vi "Dashboard Main.vi"() -> ()   [LabVIEW 2015]
uses:
  <vilib>/Utility/miscctls.llb/LVRowAndColumnTypeDef.ctl
  <vilib>/event_ctls.llb/eventvkey.ctl
  <vilib>/Rock Robotics/WPI/Dashboard/WPI_DashboardLogging Global.vi
  <vilib>/Rock Robotics/Network Tables/NT Read Numeric Array.vi
  <vilib>/Utility/config.llb/Write Key (String).vi
  <vilib>/Utility/config.llb/Write Key (I32).vi
  <vilib>/Math Plots/2D Math Plots/2D Compass/2D Compass Datatype/Public/Plot Helper (Vector).vi
  <vilib>/Utility/config.llb/NI_LVConfig.lvlib
  <vilib>/Math Plots/2D Math Plots/2D Compass/2D Compass Datatype/2D Compass Datatype.lvclass
panel:
  out "Camera Image 2":T1(plugin-control)
  in  "Switch Cams":bool
  in  "TCP":refnum<k5>
  in  "Rec Mode":enum32{"Stop", "Record", "Playback"}(radio)
  in  "Vision":u16(ring) items=["Camera Off", "USB Camera SW", "USB Camera HW", "IP Camera"]
  out "Camera IP":string
  out "Image Message":string="Timeout in Camera Communications"
  in  "Dashboard Tab":T2(tab)
  out "Gyro":dbl(knob) scale=0.0..360.0
  in  "Select Auto":string(combo)="just over defense in front"
  out "NT Connection":bool
  in  "Camera Settings":T3={"Frame Rate"=30, "Compression"=30, "Size"=1} {"Frame Rate" scale=1.0..30.0; "Size" items=["640x480", "320x240", "160x120"]}
  out "MotorChart R":cluster{"Numeric":dbl, "Numeric":dbl}(graph)
  out "MotorChart L":T4(graph)
  out "MotorSliders R":cluster{"MotorSlide1":dbl, "MotorSlide2":dbl} {"MotorSlide2" scale=-1.0..1.0 scale format="%#_2e"; "MotorSlide1" scale=-1.0..1.0 scale format="%#_2e"}
  out "MotorSliders L":T5 {"MotorSlide4 2" scale=0.0..14.0 scale format="%#_2e"; "MotorSlide2" scale=-1.0..1.0 scale format="%#_2e"; "MotorSlide1" scale=-1.0..1.0 scale format="%#_2e"}
  out "JS1 Z":dbl(slide) scale=-1.0..1.0 scale format="%#_2e"
  out "JS1 Graph":cluster{"X":dbl, "Y":dbl}[](graph)
  out "JS1 Buttons":T6
  out "JS2 Z":dbl(slide) scale=-1.0..1.0 scale format="%#_2e"
  out "JS2 Graph":cluster{"X":dbl, "Y":dbl}[](graph)
  out "JS2 Buttons":T6
  out "Mode":T7(ring)=enum."Auto Disabled"
  in  "DB Camera Config":bool
  out "fps":dbl format="%#.1g"
  out "Mbps":dbl format="%#.1g"
  out "Mbps LED":bool
  in  "DB/String 9":string
  in  "DB/String 8":string
  in  "DB/String 7":string
  in  "DB/String 6":string
  in  "DB/String 5":string
  in  "DB/String 4":string
  in  "DB/String 3":string
  in  "DB/String 2":string
  in  "DB/String 1":string
  in  "DB/String 0":string
  in  "DB/Slider 0":dbl(slide) scale=0.0..5.0
  in  "DB/Slider 1":dbl(slide) scale=0.0..5.0
  in  "DB/Slider 2":dbl(slide) scale=0.0..5.0
  in  "DB/Slider 3":dbl(slide) scale=0.0..5.0
  out "DB/LED 3":bool
  out "DB/LED 2":bool
  out "DB/LED 1":bool
  out "DB/LED 0":bool
  in  "DB/Button 3":bool
  in  "DB/Button 2":bool
  in  "DB/Button 1":bool
  in  "DB/Button 0":bool caption="New Name"
  in  "AutoMode":dbl
  in  "ClawUPDownSensitivity":dbl(slide)=0.45 step=0.025 scale=0.0..1.0
  in  "HookSensitivity":dbl(slide)=0.1 step=0.025 scale=0.0..1.0
  in  "ElevatorSensitivity":dbl(slide)=0.8500000000000001 step=0.025 scale=0.0..1.0
  in  "ClappySensitivity":dbl(slide)=0.8500000000000001 step=0.025 scale=0.0..1.0
  in  "Elevator Encoder Re-Set":bool
  in  "Elevator Height":dbl(slide) scale=0.0..7.0
  out "Manual Enabled":bool
  out "Joystick Invert":bool
  in  "F/B Invert":bool
  in  "TurningSensitivity":dbl(slide)=0.75 step=0.025 scale=0.0..1.0
  in  "ForwardSensitivity":dbl(slide)=0.8500000000000001 step=0.025 scale=0.0..1.0
  in  "Test Slider":dbl(slide) scale=0.0..100.0 scale format="%#_3g"
  in  "On/Off":bool caption="Solenoid"
  in  "Test Name":u16(ring) items=["Select the test to run..."]
  in  "Test Tree":string(tree)
  in  "Motor":cluster{"Value":dbl, "Enable":bool} {"Value" scale=-1.0..1.0 scale format="%#_3g"}
  out "Progress":T8 {"Test Progress" scale=0.0..100.0}
  in  "Rev/Fwd":cluster{"Forward":bool, "Reverse":bool}
  in  "Test Ring":u16(ring) items=["Monochrome", "Color"]
  out "Cmd Status":string
  in  "Execute Command":bool
  in  "Command Params":string[][](table)
  in  "Command Selection":i32(listbox)
  in  "CheckList":i32(listbox)
  out "Tree":string(tree)
  out "Camera Image":T1(plugin-control)
  out "Background":bool
  # "Left"
  # "Front"
  # "Right"
  # "Battery"
  # "If both inverted,\n it isn't inverted"
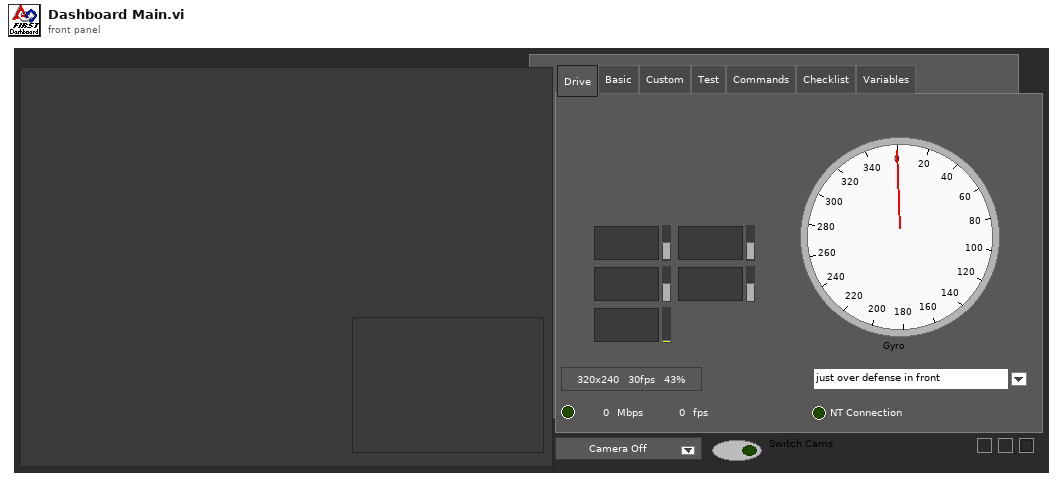
[diagram p1: front panel]
types:
  T1 = typedef "IMAQ Image.ctl" = refnum<image>
  T2 = enum32{"Drive", "Basic", "Custom", "Test", "Commands", "Checklist", "Variables"}
  T3 = cluster{"Frame Rate":i32, "Compression":i32, "Size":u16}
  T4 = cluster{"Numeric":dbl, "Numeric":dbl, "Battery V":dbl}
  T5 = cluster{"MotorSlide1":dbl, "MotorSlide2":dbl, "MotorSlide4 2":dbl}
  T6 = cluster{bool, bool, bool, bool, bool, bool, bool, bool, bool, bool, bool, bool}
  T7 = enum8{"Tele-Op Disabled", "Tele-Op Enabled", "Auto Disabled", "Auto Enabled", "Test Disabled", "Test Enabled", "Disconnected", "No Code", "E-Stop"}
  T8 = cluster{"Test Progress":u8, "Test Progress Text":string}
  T9 = typedef "Image Type" = u32
  T10 = cluster{"IDs":cluster{"RPC field ID":u16, "Unique ID":u16}, "String":string}
  T11 = enum32{"Drive", "Basic", "Custom", "Test", "Checklist", "Variables"}
  T12 = cluster{"Camera Image":refnum<vi>, "Dashboard Tab":refnum<vi>, "Background":refnum<vi>, "Vision":refnum<vi>, "Rec Mode":refnum<vi>, "Test Slider":refnum<vi>, "On/Off ":refnum<vi>, "Test Ring":refnum<vi>, "Rev/Fwd":refnum<vi>, "Test Name":refnum<vi>, "Motor":refnum<vi>, "Progress":refnum<vi>, "CheckList":refnum<vi>, "Tree":refnum<vi>, "Test Tree":refnum<vi>, "Command Params":refnum<vi>, "Command Selection":refnum<vi>, "Execute Command":refnum<vi>, "Cmd Status":refnum<vi>}
  T13 = cluster{"Error Strings":string, "Disable Counts":cluster{u16, u16}, "Rail Faults":cluster{u16, u16, u16}, "Robot IP":string, "DB Mode":u8, "Event Info":cluster{"Name":string, "Type":u8, "Number":u16, "Replay":u8}, "Camera Addr":string}
  T14 = cluster{"Storage":cluster{"Disk Free":u64, "RAM Block":u32, "RAM free":u32}, "CPU Utilization":cluster{"CPU % ISR":sgl, "CPU % Time Crit":sgl, "CPU % Timed Str":sgl, "CPU % High":sgl, "CPU % Above":sgl, "CPU % Normal":sgl, "CPU % Low":sgl}, "CAN":cluster{"% Bus Utilization":sgl, "Bus Off Cnt":u32, "TX_FIFO Full Cnt":u32, "Receive Error Cnt":u8, "Transmit Error Cnt":u8}, "HID":cluster{"HID Outputs":u32, "Rumble Low":u16, "Rumble High":u16}[]}
  T15 = cluster{"Status bits":cluster{"Test Mode":bool, "Autonomous":bool, "Enabled":bool, "Code Start":bool, "Brownout":bool, "Reserved 2":bool, "Reserved 3":bool, "E-Stop":bool}, "Code Trace":cluster{"Disabled":bool, "TeleOp":bool, "Auto":bool, "Test":bool}, "Controller Type":enum16{"unknown", "cRIO", "roboRio"}, "Code?":enum16{"unknown", "noCode", "code"}, "Battery V":dbl}
  T16 = cluster{"Control Bits":cluster{"TestMode":bool, "Autonomous":bool, "Enabled":bool, "FMS Present":bool, bool, bool, bool, "E-Stop":bool}, "Team Station ":u8, "Countdown":sgl, "Joystick Values":cluster{"Axes":dbl[], "Buttons":bool[], "POVs":i16[]}[]}
  T17 = cluster{"Axes":dbl[], "Buttons":bool[], "POVs":i16[]}[]
  T18 = cluster{"Axes":dbl[], "Buttons":bool[], "POVs":i16[]}
  T19 = cluster{"Buttons[0]":bool, "Buttons[1]":bool, "Buttons[2]":bool, "Buttons[3]":bool, "Buttons[4]":bool, "Buttons[5]":bool, "Buttons[6]":bool, "Buttons[7]":bool, "Buttons[8]":bool, "Buttons[9]":bool, "Buttons[10]":bool, "Buttons[11]":bool}
  T20 = typedef "NI_LVConfig.lvlib/Config Data RefNum.ctl" = refnum<k1>
  T21 = cluster{"Operation":enum16{"Update", "Clear"}, "Color Box":u32}[]
  T22 = typedef "eventvkey.ctl" = enum16{"ASCII", "Enter", "Return", "Shift", "Ctrl", "Alt", "Cmd", "Opt", "Caps", "NumLock", "Clear", "Break", "Up", "Down", "Left", "Right", "Insert", "Delete", "Home", "End", "PageUp", "PageDown", "Escape", "Help", "Pause", "ScrollLock", "F1", "F2", "F3", "F4", "F5", "F6", "F7", "F8", "F9", "F10", "F11", "F12", "F13", "F14", "F15", "F16", "F17", "F18", "F19", "F20", "F21", "F22", "F23", "F24", "Play", "VolumeUp", "VolumeDown", "Mute", "Two Byte Char"}
  T23 = cluster{"Image Size":bool, "Image Type":bool, "Pixel Value":bool, "ROI Information":bool, "Zoom Factor":bool}
  T24 = enum8{"Enabled", "Disabled", "Disabled and Grayed Out"}
  T25 = cluster{"Operation":enum16{"Update", "Clear"}, "Color Box":u32}
  T26 = typedef "LVRowAndColumnTypeDef.ctl" = cluster{"Row":i32, "Column":i32}
  T27 = cluster{"Shift":bool, "Ctrl":bool, "Alt":bool, "Cmd":bool, "Opt":bool}
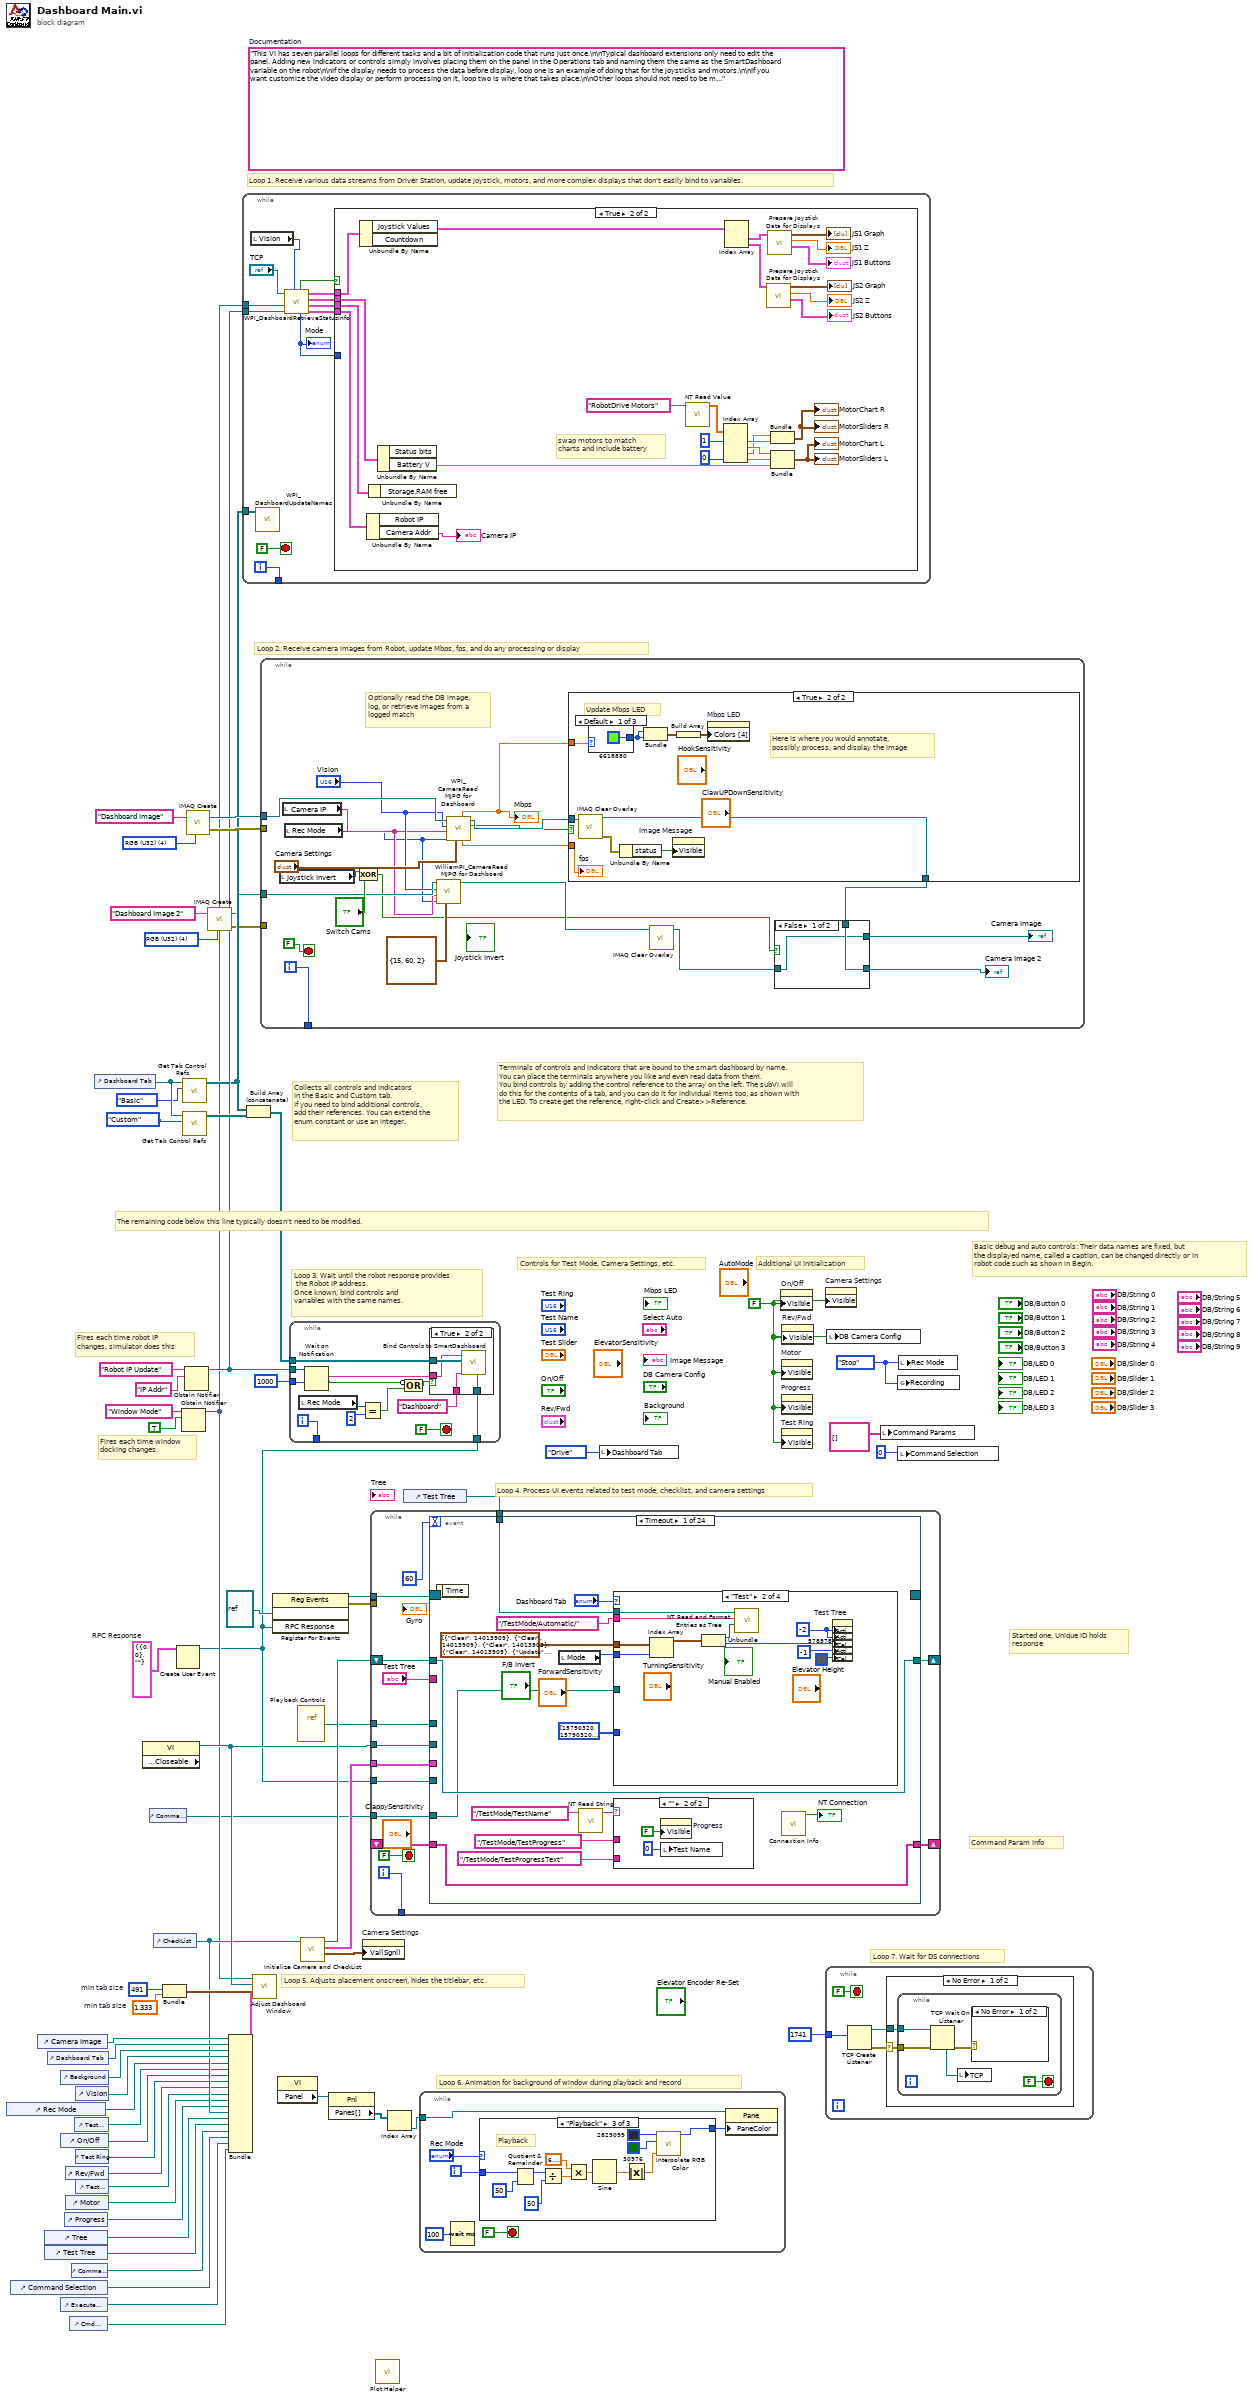
[diagram p0: block diagram]
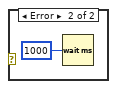
[diagram p2: hidden frame]
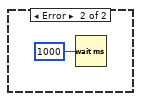
[diagram p3: hidden frame]
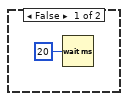
[diagram p4: hidden frame]
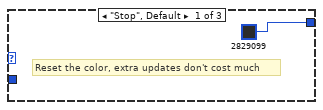
[diagram p5: hidden frame]
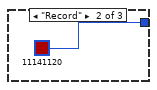
[diagram p6: hidden frame]
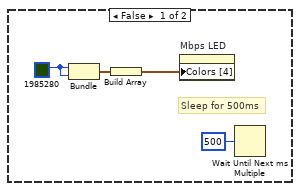
[diagram p9: hidden frame]
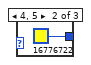
[diagram p10: hidden frame]
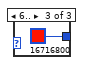
[diagram p11: hidden frame]
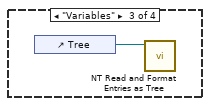
[diagram p13: hidden frame]
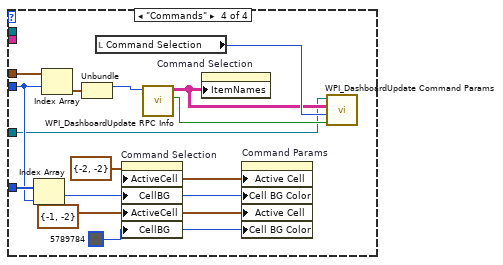
[diagram p14: hidden frame]
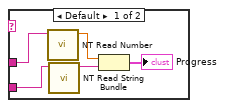
[diagram p15: hidden frame]
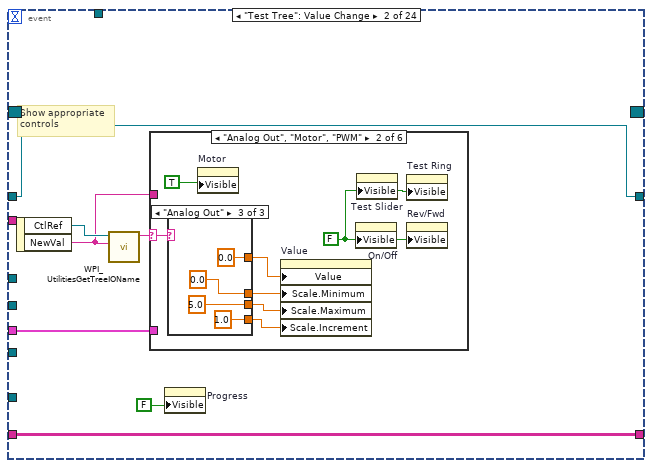
[diagram p16: hidden frame]
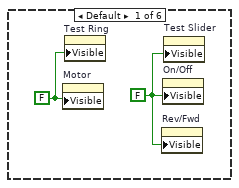
[diagram p17: hidden frame]
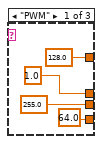
[diagram p18: hidden frame]
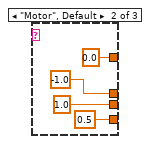
[diagram p19: hidden frame]
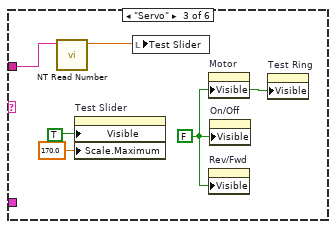
[diagram p20: hidden frame]
diagram:
  w4 = T9 4 items=["Grayscale (U8)", "Grayscale (I16)", "Grayscale (SGL)", "Complex (CSG)", "RGB (U32)", "HSL (U32)", "RGB (U64)"] ("Image Type")
  w11 = T10 {"IDs"={"RPC field ID"=0, "Unique ID"=0}, "String"=""}  # RPC Response
  w37 = 491  # min tab size
  w36 = 1.333  # min tab size
  w45 = enum32{"Stop", "Record", "Playback"}."Stop" ("Rec Mode")
  w19 = FALSE ("Visible")
  (unwired) "This VI has seven parallel loops for different tasks and a bit of initialization code that runs just once.\n\nTypical dashboard extensions only need to edit the panel. Adding new indicators or controls simply involves placing them on the panel in the Operations tab and naming them the same as the SmartDashboard variable on the robot\n\nIf the display needs to process the data before display, loop one is an example of doing that for the joysticks and motors.\n\nIf you want customize the video display or perform processing on it, loop two is where that takes place.\n\nOther loops should not need to be modified. They are pretty standard, and document the task they perform."  # Documentation
  w65 = T9 4 items=["Grayscale (U8)", "Grayscale (I16)", "Grayscale (SGL)", "Complex (CSG)", "RGB (U32)", "HSL (U32)", "RGB (U64)"] ("Image Type")
  # "Command Param Info"
  # "Started one, Unique ID holds\nresponse"
  # "Loop 7. Wait for DS connections"
  # "Basic debug and auto controls: Their data names are fixed, but\nthe displayed name, called a caption, can be changed directly or in\nrobot code such as shown in Begin."
  # "Controls for Test Mode, Camera Settings, etc."
  # "Additional UI Initialization"
  # "Loop 6. Animation for background of window during playback and record"
  # "Fires each time robot IP\nchanges, simulator does this"
  # "Fires each time window\ndocking changes."
  # "Collects all controls and indicators\nin the Basic and Custom tab.\nIf you need to bind additional controls,\nadd their references. You can extend the\nenum constant or use an integer."
  # "The remaining code below this line typically doesn't need to be modified."
  # "Loop 4. Process UI events related to test mode, checklist, and camera settings"
  # "Terminals of controls and indicators that are bound to the smart dashboard by name.\nYou can place the terminals anywhere you like and even read data from them.\nYou bind controls by adding the control reference to the array on the left. The subVI will\ndo this for the contents of a tab, and you can do it for individual items too, as shown with\nthe LED. To create get the reference, right-click and Create>>Reference."
  # "Loop 3. Wait until the robot response provides\n the Robot IP address.\nOnce known, bind controls and\nvariables with the same names."
  # "Loop 5. Adjusts placement onscreen, hides the titlebar, etc."
  # "Loop 1. Receive various data streams from Driver Station, update joystick, motors, and more complex displays that don't easily bind to variables."
  # "Loop 2. Receive camera images from Robot, update Mbps, fps, and do any processing or display"
  n1 = control-ref of="Rec Mode"() -> (w25:refnum<vi>)
  n2 = control-ref of="Command Selection"() -> (w10:refnum<vi>)
  n3 = control-ref of="Camera Image"() -> (w40:refnum<vi>)
  n4 = control-ref of="Tree"() -> (w29:refnum<vi>)
  n5 = control-ref of="Test Tree"() -> (w28:refnum<vi>)
  n6 = control-ref of="Dashboard Tab"() -> (w39:refnum<vi>)
  n7 = control-ref of="Execute Command"() -> (w12:refnum<vi>)
  n8 = control-ref of="Background"() -> (w34:refnum<vi>)
  n9 = control-ref of="On/Off"() -> (w23:refnum<vi>)
  n10 = control-ref of="Progress"() -> (w20:refnum<vi>)
  n11 = control-ref of="Rev/Fwd"() -> (w21:refnum<vi>)
  n12 = control-ref of="Motor"() -> (w26:refnum<vi>)
  n13 = control-ref of="Cmd Status"() -> (w6:refnum<vi>)
  n14 = control-ref of="Command Params"() -> (w13:refnum<vi>)
  n15 = control-ref of="Test Slider"() -> (w24:refnum<vi>)
  n16 = control-ref of="Vision"() -> (w38:refnum<vi>)
  n17 = control-ref of="Test Ring"() -> (w22:refnum<vi>)
  n18 = control-ref of="Test Name"() -> (w27:refnum<vi>)
  n19 = control-ref of="Dashboard Tab"() -> (w43:refnum<vi>)
  n20 = property class="VI" props=["Front Panel.Closeable"]() -> (reference out=w44:refnum<vi>)  [unwired: 2 in, 2 out]
  n21 = control-ref of="Command Params"() -> (w5:refnum<vi>)
  n22 = control-ref of="CheckList"() -> (w30:refnum<vi>)
  n23 = Bundle("min tab size"=w37, "min tab size"=w36) -> (w35:cluster{"min tab size":i32, "min tab size":dbl})  [unwired: 1 in]
  n24 = Create User Event(user event datatype=w11) -> (user event=w7:refnum<user-event>)  [unwired: 1 in, 1 out]
  n25 = Obtain Notifier(name (unnamed)="Window Mode", notification data type=TRUE) -> (notifier out=w16:refnum<notifier>)  [unwired: 2 in, 2 out]
  n26 = call <vilib>:"Get Tab Control Refs.vi"("Page Index"=T11."Basic" ("Dashboard Tab"), "TabControl in"=w43) -> ("ControlsOnPage"=w17:refnum<vi>[])  [unwired: 9 in]
  n27 = call <vilib>:"Get Tab Control Refs.vi"("Page Index"=T11."Custom" ("Dashboard Tab"), "TabControl in"=w43) -> ("ControlsOnPage"=w42:refnum<vi>[])  [unwired: 9 in]
  n28 = Obtain Notifier(name (unnamed)="Robot IP Update", notification data type="IP Addr" ("name (unnamed)")) -> (notifier out=w18:refnum<notifier>)  [unwired: 2 in, 2 out]
  n29 = call "IMAQ Create"("Image Name"="Dashboard Image", "Image Type"=w65) -> ("New Image"=w63:T1, "error out"=w62:errorcluster)  [unwired: 2 in, 1 out]
  n30 = call "IMAQ Create"("Image Name"="Dashboard Image 2", "Image Type"=w4) -> ("New Image"=w2:T1, "error out"=w1:errorcluster)  [unwired: 2 in, 1 out]
  n31 = Bundle("Camera Image"=w40, "Dashboard Tab"=w39, "Background"=w34, "Vision"=w38, "Rec Mode"=w25, "Test Slider"=w24, "On/Off"=w23, "Test Ring"=w22, "Rev/Fwd"=w21, "Test Name"=w27, "Motor"=w26, "Progress"=w20, "CheckList"=w30, "Tree"=w29, "Test Tree"=w28, "Command Params"=w13, "Command Selection"=w10, "Execute Command"=w12, "Cmd Status"=w6) -> (w31:T12)  [unwired: 1 in]
  n32 = while {
    tunnel: [w77] -> _
    tunnel: w18 -> [w71]
    tunnel: w17 -> [w70]
    tunnel: w16 -> [w66]
    i -> [w77]
    stop <- FALSE stop-if-true
    n33 = local read "Vision"() -> (w68:u16)
    n34 = call <vilib>:"WPI_DashboardUpdateNames.vi"("Controls on Tab"=w70) -> ()  [unwired: 11 in]
    n35 = call <vilib>:"WPI_DashboardRetrieveStatusInfo.vi"("Vision"=w68, "Binding Refnum"=w71, "Window Mode Notifier"=w66, "TCP Cnx"="TCP") -> ("Power and Errors"=w72:T13, "Robot Metrics"=w75:T14, "Status Info"=w76:T15, "Control Info"=w73:T16, "Robot Mode"=w69:T7, "Process?"=w74:bool)  [unwired: 2 in]
    "Mode" <- w69
    n36 = case shown="True" w74 {
      tunnel: w76 -> [_ w104]
      tunnel: w75 -> [_ w103]
      tunnel: w73 -> [_ w102]
      tunnel: w72 -> [_ w101]
      tunnel: w69 -> [_ _]
      frame False {
        n37 = Wait (ms)(milliseconds to wait=u32 20) -> ()  [unwired: 1 out]
      }
      frame True {
        # "swap motors to match\ncharts and include battery"
        n38 = Unbundle By Name(w102) -> ("Joystick Values"=w91:T17)  [unwired: 1 out]
        n39 = Unbundle By Name(w101) -> ("Camera Addr"=→"Camera IP":string)  [unwired: 1 out]
        n40 = Unbundle By Name(w103) -> ()  [unwired: 1 out]
        n41 = Unbundle By Name(w104) -> ("Battery V"=w92:dbl)  [unwired: 1 out]
        n42 = call-poly <vilib>:"NT Read Value.vi"("Name"="RobotDrive Motors") -> ("Numeric Array"=w80:dbl[])  [unwired: 9 in, 1 out]
        n43 = Index Array(array=w80, index #1=1, index #4=0) -> (element #1=w96:dbl, element #2=w97:dbl, element #3=w95:dbl, element #4=w100:dbl)  [unwired: 2 in]
        n44 = Index Array(array=w91) -> (element #1=w90:T18, element #2=w85:T18)  [unwired: 2 in]
        n45 = call "Prepare Joystick Data for Displays.vi"("Joystick Values"=w85) -> ("Buttons"=→"JS2 Buttons":T19, "Z Axis"=→"JS2 Z":dbl, "Cartesian Data"=→"JS2 Graph":cluster{"X axis":dbl, "X axis":dbl}[])  [unwired: 8 in]
        n46 = call "Prepare Joystick Data for Displays.vi"("Joystick Values"=w90) -> ("Buttons"=→"JS1 Buttons":T19, "Z Axis"=→"JS1 Z":dbl, "Cartesian Data"=→"JS1 Graph":cluster{"X axis":dbl, "X axis":dbl}[])  [unwired: 8 in]
        n47 = Bundle("Numeric"=w95, "Numeric"=w96) -> (→"MotorChart R" →"MotorSliders R":cluster{"Numeric":dbl, "Numeric":dbl})  [unwired: 1 in]
        n48 = Bundle("Numeric"=w97, "Numeric"=w100, "Battery V"=w92) -> (→"MotorChart L" →"MotorSliders L":T4)  [unwired: 1 in]
      }
    }
  }
  n49 = Build Array (concatenate)(w17, w42) -> (w41:refnum<vi>[])
  n50 = call "Adjust Dashboard Window.vi"("Sizing Refnums"=w31, "Size Constraints"=w35, "VI"=w44, "WIn Mode"=w16) -> ()  [unwired: 8 in]
  n51 = while {
    tunnel: w63 -> [w123]
    tunnel: w62 -> [_]
    tunnel: [w124] -> _
    tunnel: w2 -> [w109]
    tunnel: w1 -> [_]
    i -> [w124]
    stop <- FALSE stop-if-true
    # "Optionally read the DB image,\nlog, or retrieve images from a\nlogged match"
    n52 = local read "Joystick Invert"() -> (w116:bool)
    n53 = local read "Camera IP"() -> (w107:string)
    n54 = local read "Rec Mode"() -> (w106:enum32{"Stop", "Record", "Playback"})
    n55 = Exclusive Or(1:"Switch Cams", 2:w116) -> (0:w105:bool)
    n56 = call "WilliamPI_CameraRead MJPG for Dashboard.vi"("Camera Settings"=T3 {"Frame Rate"=15, "Compression"=60, "Size"=2}, "Rec Mode"=w106, "Camera IP"=w107, "Camera Mode"="Vision", "Refnum in"=w109) -> ("Refnum out"=w113:T1)  [unwired: 3 in, 3 out]
    n57 = call <vilib>:"WPI_CameraRead MJPG for Dashboard.vi"("Camera Settings"="Camera Settings", "Rec Mode"=w106, "Camera IP"=w107, "Camera Mode"="Vision", "Refnum in"=w123) -> ("Active"=w117:bool, "Refnum out"=w119:T1, "FPS"=w121:dbl, "Bandwidth (Mbps)"=w120:dbl)  [unwired: 3 in]
    "Mbps" <- w120
    n58 = case shown="True" w117 {
      tunnel: w121 -> [_ w137]
      tunnel: w120 -> [_ w136]
      tunnel: w119 -> [_ w135]
      tunnel: [_ w134] -> w115
      frame False {
        w130 = u32 1985280 ("Color Box")
        # "Sleep for 500ms"
        n59 = Bundle("Color Box"=w130, "Color Box"=w130) -> (w132:cluster{"Color Box":u32, "Color Box":u32})  [unwired: 1 out]
        n60 = Build Array(w132) -> (w131:cluster{"Color Box":u32, "Color Box":u32}[])
        n61 = property on="Mbps LED" class="Bool (strict)"("Colors [4]"=w131) -> ()  [unwired: 2 in, 2 out]
        n62 = Wait Until Next ms Multiple(millisecond multiple=u32 500) -> ()  [unwired: 1 out]
      }
      frame True {
        # "Here is where you would annotate,\npossibly process, and display the image"
        # "Update Mbps LED"
        n63 = call "IMAQ Clear Overlay"("Image"=w135) -> ("error out"=w141:errorcluster, "Image Out"=w134:T1)  [unwired: 2 in, 7 out]
        n64 = case shown="Default" w136 {
          tunnel: [u32 6618880 ("Color Box") u32 16776722 ("Color Box") u32 16716800 ("Color Box")] -> w138
          frame Default {
          }
          frame 4, 5 {
          }
          frame 6.. {
          }
        }
        n65 = Unbundle By Name(w141) -> ("status"=w142:bool)
        n66 = Bundle("Color Box"=w138, "Color Box"=w138) -> (w140:cluster{"Color Box":u32, "Color Box":u32})  [unwired: 1 out]
        n67 = property on="Image Message" class="Str"("Visible"=w142) -> ()  [unwired: 2 in, 2 out]
        n68 = Build Array(w140) -> (w139:cluster{"Color Box":u32, "Color Box":u32}[])
        n69 = property on="Mbps LED" class="Bool (strict)"("Colors [4]"=w139) -> ()  [unwired: 2 in, 2 out]
        "fps" <- w137
      }
    }
    n70 = call "IMAQ Clear Overlay"("Image"=w113) -> ("Image Out"=w112:T1)  [unwired: 2 in, 8 out]
    n71 = case shown="False" w105 {
      tunnel: w115 -> [w127 w129]
      tunnel: [w126 w129] -> w114
      tunnel: w112 -> [w126 w128]
      tunnel: [w127 w128] -> w111
      frame False {
      }
      frame True {
      }
    }
    "Camera Image" <- w114
    "Camera Image 2" <- w111
  }
  n72 = register-events(refnum<vi> refnum, w7) -> (reference out=w49:refnum<event-registration>, error out=w48:errorcluster)  [unwired: 2 in]
  n73 = property class="VI"() -> ("Panel"=w52:refnum<vi>)  [unwired: 2 in, 2 out]
  n74 = while {
    tunnel: w41 -> [w158]
    tunnel: w18 -> [w156]
    tunnel: [w154] -> _
    tunnel: u32 1000 ("milliseconds to wait") -> [w153]
    tunnel: w7 -> [w146]
    i -> [w154]
    stop <- FALSE stop-if-true
    n75 = local read "Rec Mode"() -> (w149:enum32{"Stop", "Record", "Playback"})
    n76 = Wait on Notification(notifier=w156, timeout in ms (-1)=w153) -> (notification=w155:string, timed out?=w151:bool)  [unwired: 2 in, 2 out]
    n77 = Equal?(x=w149, y=u16 2 ("Rec Mode")) -> (x = y?=w150:bool)
    n78 = Compound Arithmetic op=OR(invert w151, w150) -> (w152:bool)
    n79 = case shown="True" w152 {
      tunnel: w158 -> [_ w162]
      tunnel: w155 -> [_ w161]
      tunnel: "Dashboard" -> [_ w160]
      tunnel: w146 -> [_ w159]
      frame False {
      }
      frame True {
        n80 = call <vilib>:"Bind Controls to SmartDashboard.vi"("RPC ref"=w159, "Client Name"=w160, "Bound Control Refs"=w162, "Server IP Address"=w161) -> ()  [unwired: 8 in]
      }
    }
  }
  n81 = vi-ref "Playback Controls.vi"() -> (w50:refnum<vi>)
  n82 = call "Initialize Camera and CheckList.vi"("ListBox in"=w30) -> ("Cluster"=w56:cluster{"value":i32, "value":i32, "index":i32}, "Array"=w57:cluster{string[]}[], "File Refnum"=w55:T20)  [unwired: 8 in]
  n83 = property class="Pnl"(reference=w52) -> ("Panes[]"=w53:refnum<vi>[])  [unwired: 1 in, 2 out]
  n84 = property on="Camera Settings" class="Clust (strict)"("Val(Sgnl)"=w56) -> ()  [unwired: 2 in, 2 out]
  n85 = call-poly <vilib>:"Plot Helper.vi"() -> ()  [unwired: 4 in, 8 out]
  n86 = Index Array(array=w53) -> (element=w51:refnum<vi>)  [unwired: 1 in]
  n87 = control-ref of="Test Tree"() -> (w54:refnum<vi>)
  n88 = while {
    tunnel: w57 -> [w174]
    shift-right: [w173] -> _
    shift-left: w55 -> [w172]
    tunnel: [w171] -> _
    tunnel: w54 -> [w170]
    tunnel: w50 -> [w169]
    tunnel: w49 -> [w168]
    tunnel: w48 -> [_]
    tunnel: w44 -> [w167]
    tunnel: w7 -> [w166]
    tunnel: w5 -> [w165]
    shift-right: [w164] -> _
    shift-left: _ -> [w163]
    i -> [w171]
    stop <- FALSE stop-if-true
    n89 = event shown="[0] Timeout" {
      selector: w168 -> [_ _ _ _ _ _ _ _ _ _ _ _ _ _ _ _ _ _ _ _ _ _ _ _]
      dyn-events: [_ _ _ _ _ _ _ _ _ _ _ _ _ _ _ _ _ _ w483 _ _ _ _ _] -> _
      timeout: u32 60 ("milliseconds to wait") -> [_ _ _ _ _ _ _ _ _ _ _ _ _ _ _ _ _ _ _ _ _ _ _ _]
      tunnel: w170 -> [w187 _ _ _ _ _ _ _ _ _ _ _ _ _ _ _ _ _ _ _ _ _ _ _]
      tunnel: "Test Tree" -> [_ _ _ _ _ _ _ _ _ _ _ _ _ w446 w455 w458 w463 w472 _ _ _ _ _ _]
      tunnel: w174 -> [_ w225 _ _ _ _ _ _ _ _ _ w408 w439 _ _ _ _ _ _ _ _ _ _ _]
      tunnel: [w184 w224 w328 w334 w344 w348 w354 w366 w374 w380 w393 w407 w432 w445 w453 w457 w462 w471 w485 w501 w503 w511 w522 w527] -> w173
      tunnel: w172 -> [w184 w224 w328 w334 w344 w348 w354 w366 w374 w380 w393 w406 w432 w445 w453 w457 w462 w471 w485 w501 w503 w511 w522 w527]
      tunnel: w169 -> [_ _ _ _ _ _ _ _ _ _ _ _ _ _ _ _ _ _ w486 _ w506 _ _ _]
      tunnel: w167 -> [_ _ _ _ _ _ _ _ _ _ _ _ _ _ _ _ _ _ w481 _ _ _ _ _]
      tunnel: w166 -> [_ _ _ _ _ _ _ _ _ _ _ _ _ _ _ _ _ _ w477 _ _ _ _ _]
      tunnel: w165 -> [w179 _ _ _ _ _ w352 _ _ _ _ _ _ _ _ _ _ _ _ _ _ _ _ _]
      tunnel: [w178 w223 w327 w333 w343 w349 w350 w360 w371 w379 w392 w405 w431 w444 w452 w456 w461 w470 w476 w499 w502 w507 w515 w528] -> w164
      tunnel: w163 -> [w178 w223 w327 w333 w343 w349 w350 _ _ w379 w392 w405 w431 w444 w452 w456 w461 w470 w476 w499 w502 w507 w515 w528]
      event Timeout {
        n90 = event-data() -> ()  [unwired: 1 in, 1 out]
        n91 = local read "Mode"() -> (w181:T7)
        n92 = call <vilib>:"NT Read String.vi"("Name"="/TestMode/TestName") -> ("String"=w190:string)  [unwired: 9 in, 1 out]
        n93 = case shown="\"Test\"" "Dashboard Tab" {
          tunnel: w187 -> [_ w201 _ _]
          tunnel: "/TestMode/Automatic/" ("Name Pattern") -> [_ w200 _ _]
          tunnel: T21 [{"Operation"=enum."Clear", "Color Box"=14013909}, {"Operation"=enum."Clear", "Color Box"=14013909}, {"Operation"=enum."Clear", "Color Box"=14013909}, {"Operation"=enum."Clear", "Color Box"=14013909}, {"Operation"=enum."Update", "Color Box"=14013909}, {"Operation"=enum."Update", "Color Box"=16777215}, {"Operation"=enum."Clear", "Color Box"=14013909}, {"Operation"=enum."Clear", "Color Box"=14013909}, {"Operation"=enum."Clear", "Color Box"=14013909}] -> [_ w193 _ w210]
          tunnel: w181 -> [_ w192 _ w209]
          tunnel: u32[] [15790320, 15790320, 15790320, 15790320, 16777215, 16777215, 15790320, 15790320, 15790320] -> [_ _ _ w215]
          tunnel: w179 -> [_ _ _ w203]
          frame "Custom", Default {
          }
          frame "Test" {
            w199 = -2 ("Active Item:Row Number")
            n94 = Index Array(array=w193, index=w192) -> (element=w194:T25)
            n95 = Unbundle(w194) -> ("Operation"=w195:enum16{"Update", "Clear"}, "Color Box"=w196:u32)
            n96 = call <vilib>:"NT Read and Format Entries as Tree.vi"("Operation"=w195, "Name Pattern"=w200, "Tree Refnum"=w201) -> ()  [unwired: 7 in, 2 out]
            n97 = property on="Test Tree" class="Tree (strict)"("Active Item Row Number"=w199, "ActiveColNum"=w199, "CellBG"=w196, "Active Item Row Number"=-1 ("Active Item:Row Number"), "CellBG"=u32 5789784 ("Color Box")) -> ()  [unwired: 2 in, 2 out]
          }
          frame "Variables" {
            n98 = control-ref of="Tree"() -> (w202:refnum<vi>)
            n99 = call <vilib>:"NT Read and Format Entries as Tree.vi"("Tree Refnum"=w202) -> ()  [unwired: 9 in, 2 out]
          }
          frame "Commands" {
            w211 = u32 5789784 ("Color Box")
            w212 = T26 {"Row"=-1, "Column"=-2} ("Active Cell:Active Cell")
            w214 = T26 {"Row"=-2, "Column"=-2} ("Active Cell:Active Cell")
            n100 = Index Array(array=w215, index=w209) -> (element=w213:u32)
            n101 = Index Array(array=w210, index=w209) -> (element=w208:T25)
            n102 = Unbundle(w208) -> ("Operation"=w207:enum16{"Update", "Clear"})  [unwired: 1 out]
            n103 = local read "Command Selection"() -> (w206:i32)
            n104 = property on="Command Selection" class="MCListbox (strict)"("ActiveCell"=w214, "CellBG"=w213, "ActiveCell"=w212, "CellBG"=w211) -> ()  [unwired: 2 in, 2 out]
            n105 = call <vilib>:"WPI_DashboardUpdate RPC Info.vi"("Operation"=w207) -> ("update"=w205:bool, "commands"=w204:string[][])  [unwired: 9 in]
            n106 = property on="Command Selection" class="MCListbox (strict)"("ItemNames"=w204) -> ()  [unwired: 2 in, 2 out]
            n107 = property on="Command Params" class="Tbl (strict)"("Active Cell"=w214, "Cell BG Color"=w213, "Active Cell"=w212, "Cell BG Color"=w211) -> ()  [unwired: 2 in, 2 out]
            n108 = call <vilib>:"WPI_DashboardUpdate Command Params.vi"("Update"=w205, "NewVal"=w206, "Commands"=w204, "Param Tbl"=w203) -> ()  [unwired: 7 in, 1 out]
          }
        }
        n109 = case shown="\"\"" w190 {
          tunnel: "/TestMode/TestProgress" ("Name") -> [w217 _]
          tunnel: "/TestMode/TestProgressText" ("Name") -> [w216 _]
          frame Default {
            n110 = call <vilib>:"NT Read Number.vi"("Name"=w217) -> ("Numeric"=w218:dbl)  [unwired: 9 in, 1 out]
            n111 = call <vilib>:"NT Read String.vi"("Name"=w216) -> ("String"=w219:string)  [unwired: 9 in, 1 out]
            n112 = Bundle("Numeric"=w218, "String"=w219) -> (→"Progress":cluster{"Numeric":dbl, "String":string})  [unwired: 1 in]
          }
          frame "" {
            n113 = property on="Progress" class="Clust (strict)"("Visible"=FALSE) -> ()  [unwired: 2 in, 2 out]
            n114 = local write "Test Name"(u16 0) -> ()
          }
        }
        n115 = call <vilib>:"Connextion Info.vi"() -> ("Connected"=→"NT Connection":bool)  [unwired: 10 in, 1 out]
      }
      event "Test Tree": Value Change {
        # "Show appropriate\ncontrols"
        n116 = event-data() -> ("CtlRef"=w228:refnum<vi>, "NewVal"=w226:string)  [unwired: 1 in]
        n117 = call <vilib>:"WPI_UtilitiesGetTreeIOName.vi"("NewVal"=w226, "TreeControl in"=w228) -> ("I/O Name"=w229:string)  [unwired: 9 in]
        n118 = case shown="\"Analog Out\", \"Motor\", \"PWM\"" w229 {
          selector: w229 -> [_ w236 _ w258 w267 _]
          tunnel: w226 -> [_ _ w255 w257 _ w274]
          tunnel: w225 -> [_ _ _ _ _ w273]
          frame Default {
            w231 = FALSE ("Visible")
            w230 = FALSE ("Visible")
            n119 = property on="Motor" class="Clust (strict)"("Visible"=w230) -> ()  [unwired: 2 in, 2 out]
            n120 = property on="Test Ring" class="Ring (strict)"("Visible"=w230) -> ()  [unwired: 2 in, 2 out]
            n121 = property on="Rev/Fwd" class="Clust (strict)"("Visible"=w231) -> ()  [unwired: 2 in, 2 out]
            n122 = property on="On/Off" class="Bool (strict)"("Visible"=w231) -> ()  [unwired: 2 in, 2 out]
            n123 = property on="Test Slider" class="Slide (strict)"("Visible"=w231) -> ()  [unwired: 2 in, 2 out]
          }
          frame "Analog Out", "Motor", "PWM" {
            w237 = FALSE ("Visible")
            n124 = case shown="\"Analog Out\"" w236 {
              tunnel: [1.0 ("Value") -1.0 ("Value") 0.0 ("Value")] -> w235
              tunnel: [255.0 ("Value") 1.0 ("Value") 5.0 ("Value")] -> w234
              tunnel: [128.0 ("Value") 0.0 ("Value") 0.0 ("Value")] -> w233
              tunnel: [64.0 ("Value") 0.5 ("Value") 1.0 ("Value")] -> w232
              frame "PWM" {
              }
              frame "Motor", Default {
              }
              frame "Analog Out" {
              }
            }
            n125 = property on="Motor" class="Clust (strict)"("Visible"=TRUE) -> ()  [unwired: 2 in, 2 out]
            n126 = property on="Value" class="Slide (strict)"("Value"=w233, "Scale.Minimum"=w235, "Scale.Maximum"=w234, "Scale.Increment"=w232) -> ()  [unwired: 2 in, 2 out]
            n127 = property on="On/Off" class="Bool (strict)"("Visible"=w237) -> ()  [unwired: 2 in, 2 out]
            n128 = property on="Test Slider" class="Slide (strict)"("Visible"=w237) -> ()  [unwired: 2 in, 2 out]
            n129 = property on="Test Ring" class="Ring (strict)"("Visible"=w237) -> ()  [unwired: 2 in, 2 out]
            n130 = property on="Rev/Fwd" class="Clust (strict)"("Visible"=w237) -> ()  [unwired: 2 in, 2 out]
          }
          frame "Servo" {
            w253 = FALSE ("Visible")
            n131 = call <vilib>:"NT Read Number.vi"("Name"=w255) -> ("Numeric"=w254:dbl)  [unwired: 9 in, 1 out]
            n132 = property on="Test Slider" class="Slide (strict)"("Visible"=TRUE, "Scale.Maximum"=170.0 ("Scale.Range:Maximum")) -> ()  [unwired: 2 in, 2 out]
            n133 = local write "Test Slider"(w254) -> ()
            n134 = property on="Motor" class="Clust (strict)"("Visible"=w253) -> ()  [unwired: 2 in, 2 out]
            n135 = property on="Rev/Fwd" class="Clust (strict)"("Visible"=w253) -> ()  [unwired: 2 in, 2 out]
            n136 = property on="On/Off" class="Bool (strict)"("Visible"=w253) -> ()  [unwired: 2 in, 2 out]
            n137 = property on="Test Ring" class="Ring (strict)"("Visible"=w253) -> ()  [unwired: 2 in, 2 out]
          }
          frame "Relay", "Solenoid" {
            w256 = FALSE ("Visible")
            n138 = property on="Motor" class="Clust (strict)"("Visible"=w256) -> ()  [unwired: 2 in, 2 out]
            n139 = property on="Test Slider" class="Slide (strict)"("Visible"=w256) -> ()  [unwired: 2 in, 2 out]
            n140 = Search and Replace String(input string=w257, search string="/Value  **", replace string="/Direction") -> (result string=w263:string)  [unwired: 5 in, 3 out]
            n141 = property on="Test Ring" class="Ring (strict)"("Visible"=w256) -> ()  [unwired: 2 in, 2 out]
            n142 = call <vilib>:"NT Read String.vi"("Name"=w263) -> ("String"=w261:string)  [unwired: 9 in, 1 out]
            n143 = Equal?(x="Both directions", y=w261) -> (x = y?=w259:bool)
            n144 = Not(x=w259) -> (.not. x?=w260:bool)
            n145 = property on="Rev/Fwd" class="Clust (strict)"("Visible"=w259) -> ()  [unwired: 2 in, 2 out]
            n146 = property on="On/Off" class="Bool (strict)"("Visible"=w260, "Caption.Text"=w258) -> ()  [unwired: 2 in, 2 out]
          }
          frame "Compressor", "Digital Out" {
            w266 = FALSE ("Visible")
            # "Get direction and finish"
            n147 = property on="Motor" class="Clust (strict)"("Visible"=w266) -> ()  [unwired: 2 in, 2 out]
            n148 = property on="Test Slider" class="Slide (strict)"("Visible"=w266) -> ()  [unwired: 2 in, 2 out]
            n149 = property on="Test Ring" class="Ring (strict)"("Visible"=w266) -> ()  [unwired: 2 in, 2 out]
            n150 = property on="On/Off" class="Bool (strict)"("Visible"=TRUE, "Caption.Text"=w267) -> ()  [unwired: 2 in, 2 out]
            n151 = property on="Rev/Fwd" class="Clust (strict)"("Visible"=FALSE) -> ()  [unwired: 2 in, 2 out]
          }
          frame "Camera" {
            n152 = call <vilib>:"Get Last Path Segment.vi"("String in"=w274) -> ("String out"=w275:string)  [unwired: 10 in]
            n153 = property on="On/Off" class="Bool (strict)"("Visible"=FALSE) -> ()  [unwired: 2 in, 2 out]
            n154 = property on="Motor" class="Clust (strict)"("Visible"=FALSE) -> ()  [unwired: 2 in, 2 out]
            n155 = property on="Rev/Fwd" class="Clust (strict)"("Visible"=FALSE) -> ()  [unwired: 2 in, 2 out]
            n156 = case shown="\"White Balance  **\"" w275 {
              tunnel: w274 -> [w281 w290 w299 w308 w317 _ w323]
              tunnel: w273 -> [w279 w287 w296 w305 w314 _ _]
              frame "Size  **" {
                n157 = Index Array(array=w279) -> (element=w278:cluster{string[]})  [unwired: 1 in]
                n158 = call <vilib>:"NT Read String.vi"("Name"=w281) -> ("String"=w280:string)  [unwired: 9 in, 1 out]
                n159 = Unbundle(w278) -> (w276:string[])
                n160 = Match First String(2:w276, 3:w280) -> (0:w277:i32)  [unwired: 1 out]
                n161 = property on="Test Ring" class="Ring (strict)"("Value"=w277, "Strings []"=w276) -> ()  [unwired: 2 in, 2 out]
                n162 = property on="Test Ring" class="Ring (strict)"("Visible"=TRUE) -> ()  [unwired: 2 in, 2 out]
                n163 = property on="Test Slider" class="Slide (strict)"("Visible"=FALSE) -> ()  [unwired: 2 in, 2 out]
              }
              frame "White Balance  **" {
                n164 = Index Array(array=w287, index=1) -> (element=w288:cluster{string[]})
                n165 = call <vilib>:"NT Read String.vi"("Name"=w290) -> ("String"=w289:string)  [unwired: 9 in, 1 out]
                n166 = Unbundle(w288) -> (w285:string[])
                n167 = Match First String(2:w285, 3:w289) -> (0:w284:i32)  [unwired: 1 out]
                n168 = property on="Test Ring" class="Ring (strict)"("Value"=w284, "Strings []"=w285) -> ()  [unwired: 2 in, 2 out]
                n169 = property on="Test Ring" class="Ring (strict)"("Visible"=TRUE) -> ()  [unwired: 2 in, 2 out]
                n170 = property on="Test Slider" class="Slide (strict)"("Visible"=FALSE) -> ()  [unwired: 2 in, 2 out]
              }
              frame "Exposure  **" {
                n171 = Index Array(array=w296, index=2) -> (element=w297:cluster{string[]})
                n172 = call <vilib>:"NT Read String.vi"("Name"=w299) -> ("String"=w298:string)  [unwired: 9 in, 1 out]
                n173 = Unbundle(w297) -> (w293:string[])
                n174 = Match First String(2:w293, 3:w298) -> (0:w294:i32)  [unwired: 1 out]
                n175 = property on="Test Ring" class="Ring (strict)"("Value"=w294, "Strings []"=w293) -> ()  [unwired: 2 in, 2 out]
                n176 = property on="Test Ring" class="Ring (strict)"("Visible"=TRUE) -> ()  [unwired: 2 in, 2 out]
                n177 = property on="Test Slider" class="Slide (strict)"("Visible"=FALSE) -> ()  [unwired: 2 in, 2 out]
              }
              frame "Exposure Priority  **" {
                n178 = Index Array(array=w305, index=3) -> (element=w306:cluster{string[]})
                n179 = call <vilib>:"NT Read String.vi"("Name"=w308) -> ("String"=w307:string)  [unwired: 9 in, 1 out]
                n180 = Unbundle(w306) -> (w302:string[])
                n181 = Match First String(2:w302, 3:w307) -> (0:w303:i32)  [unwired: 1 out]
                n182 = property on="Test Ring" class="Ring (strict)"("Value"=w303, "Strings []"=w302) -> ()  [unwired: 2 in, 2 out]
                n183 = property on="Test Ring" class="Ring (strict)"("Visible"=TRUE) -> ()  [unwired: 2 in, 2 out]
                n184 = property on="Test Slider" class="Slide (strict)"("Visible"=FALSE) -> ()  [unwired: 2 in, 2 out]
              }
              frame "Color Enable  **" {
                n185 = Index Array(array=w314, index=4) -> (element=w315:cluster{string[]})
                n186 = call <vilib>:"NT Read String.vi"("Name"=w317) -> ("String"=w316:string)  [unwired: 9 in, 1 out]
                n187 = Unbundle(w315) -> (w311:string[])
                n188 = Match First String(2:w311, 3:w316) -> (0:w312:i32)  [unwired: 1 out]
                n189 = property on="Test Ring" class="Ring (strict)"("Value"=w312, "Strings []"=w311) -> ()  [unwired: 2 in, 2 out]
                n190 = property on="Test Ring" class="Ring (strict)"("Visible"=TRUE) -> ()  [unwired: 2 in, 2 out]
                n191 = property on="Test Slider" class="Slide (strict)"("Visible"=FALSE) -> ()  [unwired: 2 in, 2 out]
              }
              frame Default {
                n192 = property on="Test Ring" class="Ring (strict)"("Visible"=FALSE) -> ()  [unwired: 2 in, 2 out]
                n193 = property on="Test Slider" class="Slide (strict)"("Visible"=FALSE) -> ()  [unwired: 2 in, 2 out]
              }
              frame "Brightness  **", "Color Level  **", "Compression  **", "FPS  **", "Sharpness  **" {
                n194 = call <vilib>:"NT Read Number.vi"("Name"=w323) -> ("Numeric"=w322:dbl)  [unwired: 9 in, 1 out]
                n195 = local write "Test Slider"(w322) -> ()
                n196 = property on="Test Slider" class="Slide (strict)"("Visible"=TRUE, "Scale.Maximum"=100.0 ("Scale.Range:Maximum")) -> ()  [unwired: 2 in, 2 out]
                n197 = property on="Test Ring" class="Ring (strict)"("Visible"=FALSE) -> ()  [unwired: 2 in, 2 out]
              }
            }
          }
        }
        n198 = property on="Progress" class="Clust (strict)"("Visible"=FALSE) -> ()  [unwired: 2 in, 2 out]
      }
      event "Test Name": Mouse Enter {
        # "Populate the ring with the list of tests"
        n199 = event-data() -> ()  [unwired: 1 in, 1 out]
        n200 = call <vilib>:"NT Read String Array.vi"("Name"="/TestMode/TestList") -> ("String Array"=w332:string[])  [unwired: 9 in, 1 out]
        n201 = Build Array (concatenate)("Select the test to run...", w332) -> (w331:string[])
        n202 = property on="Test Name" class="Ring (strict)"("Strings []"=w331) -> ()  [unwired: 2 in, 2 out]
      }
      event "Test Name": Value Change {
        w335 = FALSE ("Visible")
        # "Tell the robot the test name to run"
        n203 = event-data() -> ("NewVal"=w339:u16)  [unwired: 1 in]
        n204 = property on="Test Name" class="Ring (strict)"() -> ("Strings []"=w340:string[])  [unwired: 2 in, 2 out]
        n205 = local write "Progress"(T8 {"Test Progress"=0, "Test Progress Text"=""} ("Progress")) -> ()
        n206 = Index Array(array=w340, index=w339) -> (element=w338:string)
        n207 = call <vilib>:"NT Write String.vi"("String"=w338, "Name"="/TestMode/TestName") -> ()  [unwired: 9 in, 1 out]
        n208 = property on="Progress" class="Clust (strict)"("Visible"=TRUE) -> ()  [unwired: 2 in, 2 out]
        n209 = property on="Motor" class="Clust (strict)"("Visible"=w335) -> ()  [unwired: 2 in, 2 out]
        n210 = property on="Test Slider" class="Slide (strict)"("Visible"=w335) -> ()  [unwired: 2 in, 2 out]
        n211 = property on="On/Off" class="Bool (strict)"("Visible"=w335) -> ()  [unwired: 2 in, 2 out]
        n212 = property on="Rev/Fwd" class="Clust (strict)"("Visible"=w335) -> ()  [unwired: 2 in, 2 out]
        n213 = property on="Test Ring" class="Ring (strict)"("Visible"=w335) -> ()  [unwired: 2 in, 2 out]
      }
      event "Select Auto": Mouse Enter {
        # "Populate the combo box with the list of autonomous options"
        n214 = event-data() -> ()  [unwired: 1 in, 1 out]
        n215 = call <vilib>:"NT Read String Array.vi"("Name"="Auto List") -> ("String Array"=w342:string[])  [unwired: 9 in, 1 out]
        n216 = property on="Select Auto" class="CmbBox"("Strings[]"=w342) -> ()  [unwired: 2 in, 2 out]
      }
      event "Select Auto": Value Change {
        # "User modified the Auto Selection. Write to NT variable so robot knows."
        n217 = event-data() -> ("NewVal"=w346:string)  [unwired: 1 in]
        n218 = call <vilib>:"NT Write String.vi"("String"=w346, "Name"="Auto Selector") -> ()  [unwired: 9 in, 1 out]
      }
      event "Command Selection": Value Change {
        # "Get the params and show in table"
        n219 = event-data() -> ("NewVal"=w353:i32)  [unwired: 1 in]
        n220 = property on="Command Selection" class="MCListbox (strict)"() -> ("ItemNames"=w351:string[][])  [unwired: 2 in, 2 out]
        n221 = call <vilib>:"WPI_DashboardUpdate Command Params.vi"("NewVal"=w353, "Commands"=w351, "Param Tbl"=w352) -> ()  [unwired: 8 in, 1 out]
      }
      event "Execute Command": Value Change {
        # "Started one, Unique ID holds\nresponse"
        n222 = event-data() -> ()  [unwired: 1 in, 1 out]
        n223 = property on="Command Selection" class="MCListbox (strict)"() -> ("ItemNames"=w365:string[][])  [unwired: 2 in, 2 out]
        n224 = Index Array(array=w365, index (row)="Command Selection", index (col)=0) -> (element=w363:string)
        n225 = call <vilib>:"Invoke Commands.vi"("Command Params"="Command Params", "Function Name"=w363) -> ("Params"=w359:u8, "Started"=w358:bool)  [unwired: 7 in, 1 out]
        n226 = Array Subset(array="Command Params", length (row)=w359) -> (w360:string[][])  [unwired: 3 in]
        n227 = Select(t="Executing" ("Cmd Status"), s=w358, f="" ("Cmd Status")) -> (s? t:f=→"Cmd Status":string)
      }
      event "Command Selection": Double Click {
        n228 = event-data() -> ("Row"=w375:i32)  [unwired: 1 in]
        n229 = property on="Command Selection" class="MCListbox (strict)"() -> ("ItemNames"=w378:string[][])  [unwired: 2 in, 2 out]
        n230 = local read "Command Params"() -> (w373:string[][])
        n231 = Index Array(array=w378, index (row)=w375, index (col)=0) -> (element=w376:string)
        n232 = call <vilib>:"Invoke Commands.vi"("Command Params"=w373, "Function Name"=w376) -> ("Params"=w372:u8, "Started"=w367:bool)  [unwired: 7 in, 1 out]
        n233 = Array Subset(array=w373, length (row)=w372) -> (w371:string[][])  [unwired: 3 in]
        n234 = Select(t="Executing" ("Cmd Status"), s=w367, f="" ("Cmd Status")) -> (s? t:f=w368:string)
        n235 = local write "Cmd Status"(w368) -> ()
      }
      event "CheckList": Double Click {
        # "Shift clears all"
        # "Update symbols on the listbox"
        n236 = event-data() -> ("PlatMods.Shift"=w381:bool, "Row"=w383:i32)  [unwired: 1 in]
        n237 = case shown="True" w381 {
          tunnel: w383 -> [w387 _]
          tunnel: 1 -> [w386 _]
          frame False {
            n238 = property on="CheckList" class="LstBox (strict)"() -> ("Item Symbols"=w385:i32[])  [unwired: 2 in, 2 out]
            n239 = Replace Array Subset(array=w385, new element=w386, index=w387) -> (w384:i32[])
            n240 = property on="CheckList" class="LstBox (strict)"("Item Symbols"=w384) -> ()  [unwired: 2 in, 2 out]
          }
          frame True {
            w388 = 0 ("Top Row")
            n241 = property on="CheckList" class="LstBox (strict)"() -> ("Number of Rows"=w390:u32)  [unwired: 2 in, 2 out]
            n242 = Initialize Array(0, w390) -> (w389:i32[])
            n243 = property on="CheckList" class="LstBox (strict)"("Top Row"=w388, "Value"=w388, "Item Symbols"=w389) -> ()  [unwired: 2 in, 2 out]
          }
        }
      }
      event "CheckList": Key Down {
        # "Update symbols on the listbox\nLeft and right keys check and uncheck"
        n244 = event-data() -> ("VKey"=w395:T22)  [unwired: 1 in]
        n245 = case shown="\"Left\", \"Right\"" w395 {
          selector: w395 -> [w400 _]
          tunnel: eventvkey."Left" ("VKey") -> [w398 _]
          frame "Left", "Right" {
            n246 = Equal?(x=w398, y=w400) -> (x = y?=w399:bool)
            n247 = Select(t=0, s=w399, f=1) -> (s? t:f=w401:i32)
            n248 = property on="CheckList" class="LstBox (strict)"() -> ("Item Symbols"=w404:i32[])  [unwired: 2 in, 2 out]
            n249 = Replace Array Subset(array=w404, new element=w401, index="CheckList") -> (w403:i32[])
            n250 = property on="CheckList" class="LstBox (strict)"("Item Symbols"=w403) -> ()  [unwired: 2 in, 2 out]
          }
          frame Default {
          }
        }
      }
      event "DB Camera Config": Value Change {
        # "Show or hide the cluster of controls, store in ini file"
        n251 = event-data() -> ("NewVal"=w409:bool)  [unwired: 1 in]
        n252 = case shown="False" w409 {
          tunnel: w408 -> [w418 _]
          tunnel: [w411 w429] -> w407
          tunnel: w406 -> [w410 w429]
          frame False {
            w425 = "Camera"
            w428 = FALSE ("Visible")
            n253 = local read "Camera Settings"() -> (w417:T3)
            n254 = Index Array(array=w418) -> (element=w421:cluster{string[]})  [unwired: 1 in]
            n255 = Unbundle(w417) -> ("Frame Rate"=w416:i32, "Compression"=w415:i32, "Size"=w419:u16)
            n256 = Unbundle(w421) -> (w420:string[])
            n257 = Index Array(array=w420, index=w419) -> (element=w414:string)
            n258 = call-poly <vilib>:"Write Key.vi"("section"=w425, "value"=w414, "key"="Size", "refnum"=w410) -> ("refnum out"=w427:T20)  [unwired: 2 in, 5 out]
            n259 = call-poly <vilib>:"Write Key.vi"("section"=w425, "value"=w416, "key"="FrameRate", "refnum"=w427) -> ("refnum out"=w426:T20)  [unwired: 1 in, 6 out]
            n260 = property on="Camera Settings" class="Clust (strict)"("Visible"=w428) -> ()  [unwired: 2 in, 2 out]
            n261 = local write "DB Camera Config"(w428) -> ()
            n262 = call-poly <vilib>:"Write Key.vi"("section"=w425, "value"=w415, "key"="Compression", "refnum"=w426) -> ("refnum out"=w412:T20)  [unwired: 1 in, 6 out]
            n263 = call <vilib>:"Close Config Data.vi"("refnum"=w412) -> ("file path"=w413:path)  [unwired: 2 in, 8 out]
            n264 = call <vilib>:"Open Config Data.vi"("configuration file path"=w413) -> ("refnum"=w411:T20)  [unwired: 8 in, 2 out]
          }
          frame True {
            n265 = property on="Camera Settings" class="Clust (strict)"("Visible"=TRUE) -> ()  [unwired: 2 in, 2 out]
          }
        }
      }
      event "Camera Settings": Value Change {
        # "Update summary string when any elements of DB camera change"
        n266 = event-data() -> ("NewVal"=w443:T3)  [unwired: 1 in]
        n267 = Index Array(array=w439) -> (element=w438:cluster{string[]})  [unwired: 1 in]
        n268 = Unbundle(w443) -> ("Frame Rate"=w434:i32, "Compression"=w433:i32, "Size"=w436:u16)
        n269 = Unbundle(w438) -> (w437:string[])
        n270 = Index Array(array=w437, index=w436) -> (element=w435:string)
        n271 = Format Into String(format string="%s   %dfps   %d%%", w435, w434, w433) -> (resulting string=w440:string)  [unwired: 2 in, 1 out]
        n272 = Build Array(w440) -> (w441:string[])
        n273 = property on="DB Camera Config" class="Bool (strict)"("Strings [4]"=w441) -> ()  [unwired: 2 in, 2 out]
      }
      event "Motor.Enable": Value Change {
        # "When the test mode otor enable helper is set, update that\ntree row item's value"
        n274 = event-data() -> ("NewVal"=w450:bool)  [unwired: 1 in]
        n275 = Unbundle("Motor") -> ("Value"=w449:dbl)  [unwired: 1 out]
        n276 = Select(t=w449, s=w450, f=0.0) -> (s? t:f=w447:dbl)
        n277 = call <vilib>:"NT Write Number.vi"("Numeric"=w447, "Name"=w446) -> ()  [unwired: 9 in, 1 out]
      }
      event "Test Slider": Value Change {
        # "When the test mode slider helper is set, update that\ntree row item's value"
        n278 = event-data() -> ("NewVal"=w454:dbl)  [unwired: 1 in]
        n279 = call <vilib>:"NT Write Number.vi"("Numeric"=w454, "Name"=w455) -> ()  [unwired: 9 in, 1 out]
      }
      event "On/Off": Value Change {
        # "When the test mode on/off helper value is set, update that\ntree row item's value"
        n280 = event-data() -> ("NewVal"=w460:bool)  [unwired: 1 in]
        n281 = Boolean To (0,1)(Boolean=w460) -> (0, 1=w459:i16)
        n282 = call <vilib>:"NT Write Number.vi"("Numeric"=w459, "Name"=w458) -> ()  [unwired: 9 in, 1 out]
      }
      event "Rev/Fwd": Value Change {
        # "When the test mode helper value for relays is set, update that\ntree row item's value"
        n283 = event-data() -> ("NewVal.Forward"=w469:bool, "NewVal.Reverse"=w468:bool)  [unwired: 1 in]
        n284 = Boolean To (0,1)(Boolean=w469) -> (0, 1=w465:i16)
        n285 = Boolean To (0,1)(Boolean=w468) -> (0, 1=w467:i16)
        n286 = Negate(x=w467) -> (-x=w466:i16)
        n287 = Add(x=w465, y=w466) -> (x+y=w464:i16)
        n288 = call <vilib>:"NT Write Number.vi"("Numeric"=w464, "Name"=w463) -> ()  [unwired: 9 in, 1 out]
      }
      event "Test Ring": Value Change {
        # "When a test mode helper value is selected from the ring,\nset the tree item's variable to the string value"
        n289 = event-data() -> ("NewVal"=w474:u16)  [unwired: 1 in]
        n290 = property on="Test Ring" class="Ring (strict)"() -> ("Strings []"=w475:string[])  [unwired: 2 in, 2 out]
        n291 = Index Array(array=w475, index=w474) -> (element=w473:string)
        n292 = call <vilib>:"NT Write String.vi"("String"=w473, "Name"=w472) -> ()  [unwired: 9 in, 1 out]
      }
      event "Rec Mode": Value Change {
        # "Update globals for recording mode and path to read log from.\nClear when logging and let NetworkTables set path for vision to\nuse."
        n293 = event-data() -> ("NewVal"=w487:enum32{"Stop", "Record", "Playback"})  [unwired: 1 in]
        n294 = global write "WPI_DashboardLogging Global.vi" "Logging Filename"(path "") -> ()
        n295 = global write "WPI_DashboardLogging Global.vi" "Recording"(w487) -> ()
        n296 = case shown="\"Playback\"" w487 {
          tunnel: w486 -> [_ w489 w498]
          tunnel: [_ _ w497] -> w483
          tunnel: [_ _ w496] -> _
          tunnel: w481 -> [_ _ w494]
          tunnel: cluster{i32, i32} {-250, 170} -> [_ _ w493]
          tunnel: [_ _ T23 {"Image Size"=TRUE, "Image Type"=TRUE, "Pixel Value"=TRUE, "ROI Information"=TRUE, "Zoom Factor"=FALSE} ("Image Information Shown:All Elements")] -> w479
          tunnel: [_ _ TRUE ("Zoom Factor")] -> w478
          tunnel: w477 -> [_ _ w490]
          frame Default {
          }
          frame "Stop", "Record" {
            # "Place Window too"
            n297 = invoke class="VI" method="FP.Close"(reference=w489) -> (reference out=w488:refnum<vi>)  [unwired: 2 in, 2 out]
            n298 = invoke class="VI" method="Abort VI"(reference=w488) -> ()  [unwired: 2 in, 3 out]
          }
          frame "Playback" {
            n299 = call "Open Playback Panel.vi"("Offset"=w493, "DB VI Ref"=w494, "Playback in"=w498) -> ("Playback out"=w495:refnum<vi>)  [unwired: 8 in]
            n300 = register-events(w495, w490) -> (reference out=w497:refnum<event-registration>, error out=w496:errorcluster)  [unwired: 2 in]
          }
        }
        n301 = property on="Camera Image" class="ImageControl"("Image Information Shown"=w479, "Image Information Visible"=w478) -> ()  [unwired: 2 in, 2 out]
        n302 = call <vilib>:"WPI_DashboardNT Log FieldName Cache.vi"("Operation"=enum16{"Lookup/Add", "Index", "Clear"}."Clear") -> ()  [unwired: 8 in, 3 out]
      }
      event Panel Close {
        w500 = enum32{"Stop", "Record", "Playback"}."Stop" ("Rec Mode")
        # "Playback window has been closed, abort"
        n303 = event-data() -> ()  [unwired: 1 in, 4 out]
        n304 = local write "Rec Mode"(w500) -> ()
        n305 = global write "WPI_DashboardLogging Global.vi" "Recording"(w500) -> ()
      }
      event Panel Close {
        # "Abort playback window and ourself"
        n306 = event-data() -> ()  [unwired: 1 in, 4 out]
        n307 = invoke class="VI" method="FP.Close"(reference=w506) -> (reference out=w505:refnum<vi>)  [unwired: 2 in, 2 out]
        n308 = invoke class="VI" method="Abort VI"(reference=w505) -> (error out=w504:errorcluster)  [unwired: 2 in, 2 out]
        n309 = invoke class="VI" method="Abort VI"(error in=w504) -> ()  [unwired: 2 in, 3 out]
      }
      event User Event {
        n310 = event-data() -> ("IDs"=w514:cluster{"RPC field ID":u16, "Unique ID":u16}, "String"=w513:string)  [unwired: 1 in]
        n311 = Bundle("IDs"=w514, "String"=w513) -> (w512:T10)  [unwired: 1 in]
        n312 = call <vilib>:"Retrieve RPC Response.vi"("RPC Response"=w512) -> ("Output"=w509:string[][])  [unwired: 10 in]
        n313 = Build Array (concatenate)(w507, w509) -> (w508:string[][])
        n314 = local write "Command Params"(w508) -> ()
        n315 = local write "Cmd Status"("" ("Cmd Status")) -> ()
      }
      event "Vision": Value Change {
        # "Enable/Disable Compression slider.\nHW USB is hard-coded into the camera"
        n316 = event-data() -> ("NewVal"=w521:u16)  [unwired: 1 in]
        n317 = Equal?(x=w521, y=u32 2 ("milliseconds to wait")) -> (x = y?=w519:bool)
        n318 = Select(t=T24."Disabled and Grayed Out" ("Disabled"), s=w519, f=T24."Enabled" ("Disabled")) -> (s? t:f=w516:T24)
        n319 = property on="Compression" class="Slide (strict)"("DisabledEnum"=w516) -> ()  [unwired: 2 in, 2 out]
      }
      event "Tree": Double Click {
        n320 = event-data() -> ("PlatMods"=w526:T27, "Tag"=w525:string)  [unwired: 1 in]
        n321 = Unbundle(w526) -> ("Shift"=w524:bool)  [unwired: 4 out]
        n322 = Not(x=w524) -> (.not. x?=w523:bool)
        n323 = call <vilib>:"NT Update Persistence.vi"("Persistence"=w523, "Name"=w525) -> ()  [unwired: 9 in, 1 out]
      }
    }
  }
  n324 = while {
    tunnel: w51 -> [w530]
    i -> [w533]
    stop <- FALSE stop-if-true
    n325 = Wait (ms)(milliseconds to wait=u32 100) -> ()  [unwired: 1 out]
    n326 = case shown="\"Playback\"" "Rec Mode" {
      tunnel: w533 -> [_ _ w548]
      tunnel: [u32 2829099 ("Base Color") u32 11141120 ("Target Color") w537] -> w529
      frame "Stop", Default {
        # "Reset the color, extra updates don't cost much"
      }
      frame "Record" {
      }
      frame "Playback" {
        # "Playback"
        n327 = Quotient & Remainder(x=w548, y=u32 50 ("milliseconds to wait")) -> (x-y*floor(x/y)=w544:u32)  [unwired: 1 out]
        n328 = Divide(x=w544, y=u32 50 ("milliseconds to wait")) -> (x/y=w541:dbl)
        n329 = Multiply(x=6.283185307179586, y=w541) -> (x*y=w546:dbl)
        n330 = Sine(x=w546) -> (sin(x)=w545:dbl)
        n331 = Absolute Value(x=w545) -> (abs(x)=w538:dbl)
        n332 = call "Interpolate RGB Color.vi"("Proportion"=w538, "Target Color"=u32 30976, "Base Color"=u32 2829099) -> ("Result Color"=w537:u32)  [unwired: 8 in]
      }
    }
    n333 = property class="Pane"(reference=w530, "PaneColor"=w529) -> ()  [unwired: 1 in, 2 out]
  }
  n334 = local write "Dashboard Tab"(T2."Drive" ("Dashboard Tab")) -> ()
  n335 = property on="On/Off" class="Bool (strict)"("Visible"=w19) -> ()  [unwired: 2 in, 2 out]
  n336 = property on="Motor" class="Clust (strict)"("Visible"=w19) -> ()  [unwired: 2 in, 2 out]
  n337 = property on="Progress" class="Clust (strict)"("Visible"=w19) -> ()  [unwired: 2 in, 2 out]
  n338 = property on="Test Ring" class="Ring (strict)"("Visible"=w19) -> ()  [unwired: 2 in, 2 out]
  n339 = property on="Rev/Fwd" class="Clust (strict)"("Visible"=w19) -> ()  [unwired: 2 in, 2 out]
  n340 = property on="Camera Settings" class="Clust (strict)"("Visible"=w19) -> ()  [unwired: 2 in, 2 out]
  n341 = while {
    tunnel: u16 1741 ("timeout ms (25000)") -> [w550]
    stop <- FALSE stop-if-true
    n342 = TCP Create Listener(10:w550) -> (0:w549:errorcluster, 3:w551:refnum<k5>)  [unwired: 4 in, 1 out]
    n343 = case shown="No Error" w549 {
      selector: w549 -> [w553 _]
      tunnel: w551 -> [w554 _]
      frame No Error {
        n344 = while {
          tunnel: w554 -> [w557]
          tunnel: w553 -> [w556]
          stop <- FALSE stop-if-true
          n345 = TCP Wait On Listener(8:w556, 11:w557) -> (0:w558:errorcluster, 4:w559:refnum<k5>)  [unwired: 2 in, 3 out]
          n346 = local write "TCP"(w559) -> ()
          n347 = case shown="No Error" w558 {
            frame No Error {
            }
            frame Error {
              n348 = Wait (ms)(milliseconds to wait=u32 1000) -> ()  [unwired: 1 out]
            }
          }
        }
      }
      frame Error {
        n349 = Wait (ms)(milliseconds to wait=u32 1000) -> ()  [unwired: 1 out]
      }
    }
  }
  n350 = local write "DB Camera Config"(w19) -> ()
  n351 = local write "Command Params"(string[][] [] ("Command Params")) -> ()
  n352 = global write "WPI_DashboardLogging Global.vi" "Recording"(w45) -> ()
  n353 = local write "Command Selection"(u16 0 ("milliseconds to wait")) -> ()
  n354 = local write "Rec Mode"(w45) -> ()
